vi "IMAQ_Attribute2Control_U32.vi"(3 "error in (no error)":errorcluster, 4 "IMAQ Attribute":variant, 5 "Refnum (U32)":refnum<vi>) -> (0 "error out":errorcluster, 1 "dup IMAQ Attribute":variant)   [LabVIEW 2012, in "HGF_VisionTools.lvlib"]
doc: "This Polymorphic VI set IMAQ control properties of type I64 according to variant inputp value and its attribute."
uses:
  HGF_VisionTools.lvlib
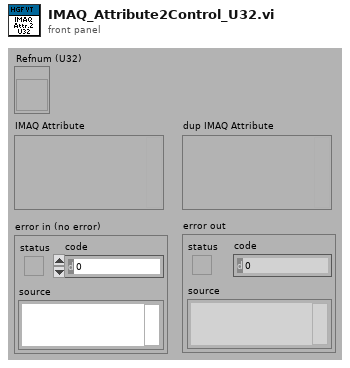
[diagram p1: front panel]
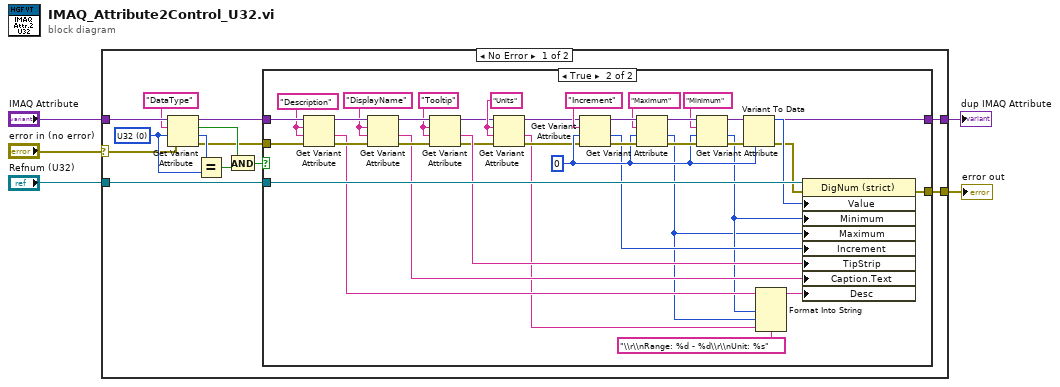
[diagram p0: block diagram]
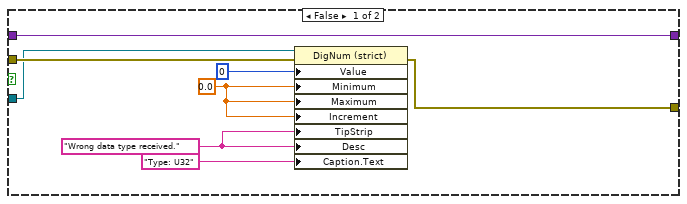
[diagram p2: hidden frame]
diagram:
  n1 = case shown="No Error" "error in (no error)" {
    selector: "error in (no error)" -> [w11 w65]
    tunnel: "IMAQ Attribute" -> [w18 w64]
    tunnel: "Refnum (U32)" -> [w8 _]
    tunnel: [w7 w65] -> w2
    tunnel: [w6 w64] -> w1
    frame No Error {
      w15 = u32 0 items=["U32", "I64", "DBL", "String", "Enum", "Bool", "Command"] ("Type")
      n2 = Get Variant Attribute(Variant=w18, name="DataType", default value (empty Variant)=w15, error in=w11) -> (duplicate Variant=w10:variant, found=w14:bool, value=w16:u32, error out=w9:errorcluster)
      n3 = Equal?(x=w16, y=w15) -> (x = y?=w13:bool)
      n4 = And(x=w14, y=w13) -> (x .and. y?=w12:bool)
      n5 = case shown="True" w12 {
        tunnel: w10 -> [w26 w63]
        tunnel: w9 -> [w22 w62]
        tunnel: w8 -> [w21 w61]
        tunnel: [w20 w40] -> w7
        tunnel: [w26 w39] -> w6
        frame False {
          w24 = "Wrong data type received." ("Tip Strip")
          w25 = 0.0 ("Value")
          n6 = property class="DigNum (strict)"(reference=w21, error in=w22, "Value"=i64 0, "Minimum"=w25, "Maximum"=w25, "Increment"=w25, "TipStrip"=w24, "Desc"=w24, "Caption.Text"="Type: U32") -> (error out=w20:errorcluster)  [unwired: 1 out]
        }
        frame True {
          w32 = "Units" ("name")
          w46 = u32 0 ("Value")
          w43 = "Tooltip" ("name")
          w37 = "Description" ("name")
          w38 = "DisplayName" ("name")
          n7 = Get Variant Attribute(Variant=w63, name=w37, default value (empty Variant)=w37, error in=w62) -> (duplicate Variant=w54:variant, value=w41:string, error out=w55:errorcluster)  [unwired: 1 out]
          n8 = Get Variant Attribute(Variant=w54, name=w38, default value (empty Variant)=w38, error in=w55) -> (duplicate Variant=w53:variant, value=w42:string, error out=w56:errorcluster)  [unwired: 1 out]
          n9 = Get Variant Attribute(Variant=w53, name=w43, default value (empty Variant)=w43, error in=w56) -> (duplicate Variant=w29:variant, value=w44:string, error out=w30:errorcluster)  [unwired: 1 out]
          n10 = Get Variant Attribute(Variant=w29, name=w32, default value (empty Variant)=w32, error in=w30) -> (duplicate Variant=w28:variant, value=w27:string, error out=w31:errorcluster)  [unwired: 1 out]
          n11 = Get Variant Attribute(Variant=w28, name="Increment", default value (empty Variant)=w46, error in=w31) -> (duplicate Variant=w59:variant, value=w45:u32, error out=w60:errorcluster)  [unwired: 1 out]
          n12 = Get Variant Attribute(Variant=w59, name="Maximum", default value (empty Variant)=w46, error in=w60) -> (duplicate Variant=w57:variant, value=w33:u32, error out=w58:errorcluster)  [unwired: 1 out]
          n13 = Get Variant Attribute(Variant=w57, name="Minimum", default value (empty Variant)=w46, error in=w58) -> (duplicate Variant=w39:variant, value=w34:u32, error out=w49:errorcluster)  [unwired: 1 out]
          n14 = Variant To Data(error in=w49, type=w46, Variant=w39) -> (data=w48:u32, error out=w47:errorcluster)
          n15 = Format Into String(format string="\\r\\nRange: %d - %d\\r\\nUnit: %s", initial string=w41, w34, w33, w27) -> (resulting string=w36:string)  [unwired: 1 in, 1 out]
          n16 = property class="DigNum (strict)"(reference=w61, error in=w47, "Value"=w48, "Minimum"=w34, "Maximum"=w33, "Increment"=w45, "TipStrip"=w44, "Caption.Text"=w42, "Desc"=w36) -> (error out=w40:errorcluster)  [unwired: 1 out]
        }
      }
    }
    frame Error {
    }
  }
  "error out" <- w2
  "dup IMAQ Attribute" <- w1
